vi "Static Error Handling.Parameters.Description.Set.vi"(10 "error description":string, 11 "error in":errorcluster) -> (1 "new offset":i32, 3 "error out":errorcluster)   [LabVIEW 2016, in "Memory Manager.lvlib" / "Static Error Handling.lvlib"]
doc: "Sets the error description of <b>error in</b>."
uses:
  Static Error Handling.lvlib
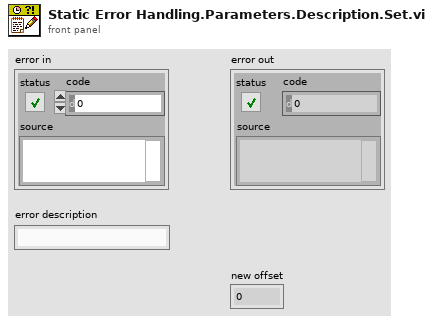
[diagram p1: front panel]
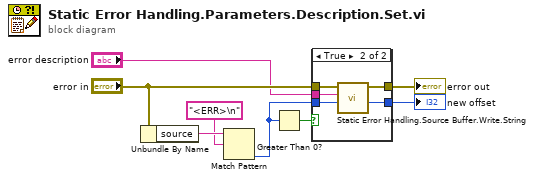
[diagram p0: block diagram]
diagram:
  n1 = Unbundle By Name("error in") -> ("source"=w8:string)
  n2 = Match Pattern(string=w8, regular expression="<ERR>\n") -> (offset past match=w2:i32)  [unwired: 1 in, 3 out]
  n3 = Greater Than 0?(x=w2) -> (x > 0?=w1:bool)
  n4 = case shown="True" w1 {
    tunnel: "error in" -> [w9 w15]
    tunnel: [w9 w14] -> w5
    tunnel: [w10 w13] -> w4
    tunnel: "error description" -> [_ w12]
    tunnel: w2 -> [w10 w11]
    frame False {
    }
    frame True {
      n5 = call "Static Error Handling.Source Buffer.Write.String.vi"("offset"=w11, "string"=w12, "error in"=w15) -> ("new offset"=w13:i32, "error out"=w14:errorcluster)  [unwired: 7 in]
    }
  }
  "error out" <- w5
  "new offset" <- w4
